vi "Update Sequencer State.vi"(8 "error in (no error)":errorcluster, 10 "Sequencer State":T1, 11 "Output Sequencer in":refnum<class "Output Sequencer.lvclass">) -> (0 "error out":errorcluster, 3 "Output Sequencer out":refnum<class "Output Sequencer.lvclass">)   [LabVIEW 2020, in "Output Sequencer.lvlib" / "Output Sequencer.lvclass"]
uses:
  Output Sequencer.lvclass
  Types/Sequencer State.ctl
  Output Sequencer.lvclass/Output Sequencer.ctl
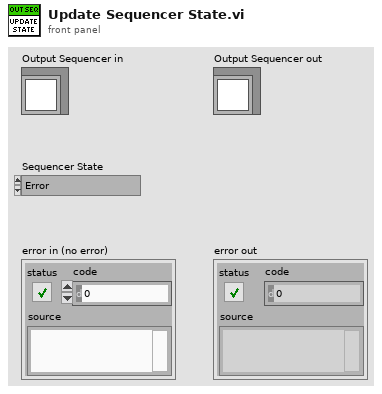
[diagram p1: front panel]
types:
  T1 = typedef "Output Sequencer.lvlib/Output Sequencer.lvclass/Sequencer State.ctl" = enum16{"Error", "Initialize", "Prepare channels", "Wait for test", "Wait for %.1f sec", "Wait for trigger", "Stop condition", "Wait for resume", "Running", "Paused", "No valid step", "Stopped"}
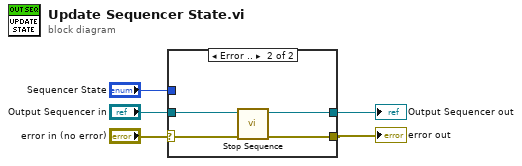
[diagram p0: block diagram]
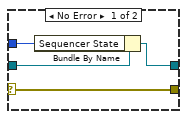
[diagram p2: hidden frame]
diagram:
  n1 = case shown="Error .." "error in (no error)" {
    selector: "error in (no error)" -> [w9 w13]
    tunnel: "Output Sequencer in" -> [w8 w12]
    tunnel: "Sequencer State" -> [w7 _]
    tunnel: [w9 w10] -> w4
    tunnel: [w6 w11] -> w5
    frame No Error {
      n2 = Bundle By Name(cluster=w8, "Sequencer State"=w7) -> (w6:refnum<class "Output Sequencer.lvclass">)
    }
    frame Error {
      n3 = call "Stop Sequence.vi"("error in (no error)"=w13, "Output Sequencer in"=w12) -> ("error out"=w10:errorcluster, "Output Sequencer out"=w11:refnum<class "Output Sequencer.lvclass">)  [unwired: 7 in, 1 out]
    }
  }
  "Output Sequencer out" <- w5
  "error out" <- w4
